vi "VCS Get Ipm Buffer Parameter.vi"(0 "axis in":cluster{"keyHandle":u32, "nodeId":u16}={"keyHandle"=0, "nodeId"=1}, 3 "error in (no error)":errorcluster) -> (5 "axis out":cluster{"keyHandle":u32, "nodeId":u16}={"keyHandle"=0, "nodeId"=1}, 6 "IPM buffer parameter":T1, 7 "maxBufferSize":u32, 8 "error out":errorcluster)   [LabVIEW 2010]
doc: "The function <B>VCS_GetIpmBufferParameter</B> reads warning borders and the max. buffer size of the data input."
uses:
  Resources/EposCmd.dll
  Resources/EposCmd64.dll
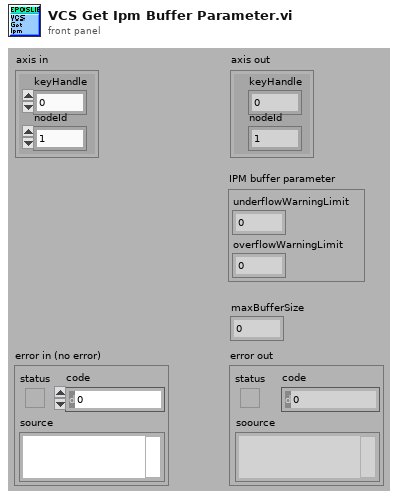
[diagram p1: front panel]
types:
  T1 = cluster{"underflowWarningLimit":u16, "overflowWarningLimit":u16}
  T2 = cluster{"pUnderflowWarningLimit":u16, "pOverflowWarningLimit":u16}
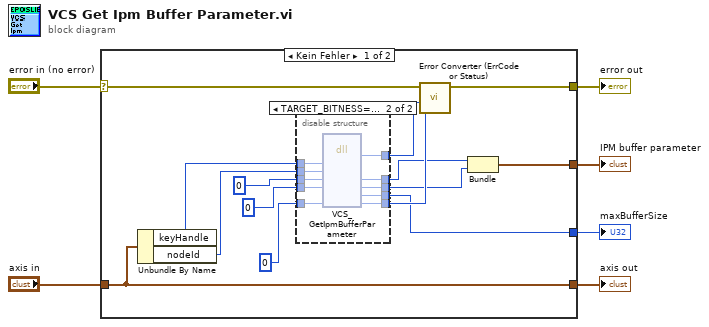
[diagram p0: block diagram]
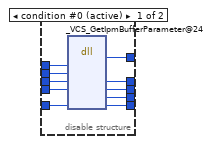
[diagram p2: hidden frame]
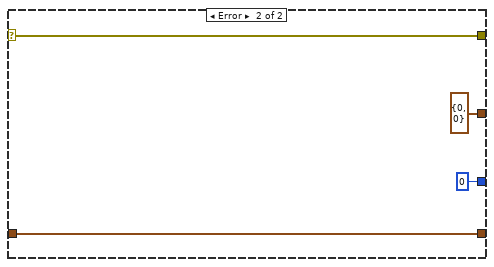
[diagram p3: hidden frame]
diagram:
  n1 = case shown="Kein Fehler" "error in (no error)" {
    selector: "error in (no error)" -> [w18 w43]
    tunnel: "axis in" -> [w20 w44]
    tunnel: [w20 w44] -> w5
    tunnel: [w19 w43] -> w4
    tunnel: [w12 u32 0 ("pMaxBufferSize")] -> w2
    tunnel: [w7 T2 {"pUnderflowWarningLimit"=0, "pOverflowWarningLimit"=0}] -> w1
    frame No Error {
      n2 = Unbundle By Name(w20) -> ("keyHandle"=w16:u32, "nodeId"=w17:u16)
      n3 = disable-structure shown="TARGET_BITNESS==64" {
        disable-tunnel: w17 -> [w30 w40]
        disable-tunnel: w16 -> [w29 w39]
        disable-tunnel: u32 0 ("pErrorCode") -> [w28 w38]
        disable-tunnel: [w27 w37] -> w14
        disable-tunnel: [w26 w36] -> w13
        disable-tunnel: [w25 w35] -> w12
        disable-tunnel: u16 0 ("pUnderflowWarningLimit") -> [w24 w34]
        disable-tunnel: u16 0 ("pOverflowWarningLimit") -> [w23 w33]
        disable-tunnel: [w22 w32] -> w9
        disable-tunnel: [w21 w31] -> w8
        frame condition #0 (active) {
          n4 = dll-call lib="C:/Sources/LabView/maxon EPOS/Resources/EposCmd.*" fn="_VCS_GetIpmBufferParameter@24"("KeyHandle"=w29, "NodeId"=w30, "pUnderflowWarningLimit"=w24, "pOverflowWarningLimit"=w23, "pErrorCode"=w28) -> (w26:i32, "pUnderflowWarningLimit"=w22:u16, "pOverflowWarningLimit"=w21:u16, "pMaxBufferSize"=w25:u32, "pErrorCode"=w27:u32)  [unwired: 6 in, 2 out]
        }
        frame condition #1 {
          n5 = dll-call lib="C:/setup/Resources/EposCmd64.*" fn="VCS_GetIpmBufferParameter" ("EposCmd.dll:_VCS_GetIpmBufferParameter@24")("KeyHandle"=w39, "NodeId"=w40, "pUnderflowWarningLimit"=w34, "pOverflowWarningLimit"=w33, "pErrorCode"=w38) -> ("Rückgabetyp"=w36:i32, "pUnderflowWarningLimit"=w32:u16, "pOverflowWarningLimit"=w31:u16, "pMaxBufferSize"=w35:u32, "pErrorCode"=w37:u32)  [unwired: 6 in, 2 out]
        }
      }
      n6 = call "Error Converter (ErrCode or Status).vi"("error code"=w14, "return type"=w13, "error in (no error)"=w18) -> ("error out"=w19:errorcluster)  [unwired: 7 in]
      n7 = Bundle("pUnderflowWarningLimit"=w9, "pOverflowWarningLimit"=w8) -> (w7:T2)  [unwired: 1 in]
    }
    frame Error {
    }
  }
  "maxBufferSize" <- w2
  "error out" <- w4
  "axis out" <- w5
  "IPM buffer parameter" <- w1
